vi "CardStatusInitial.vi"(7 "Action":enum16{"Initial", "Write", "Read", "Release"}(ring)=enum."Release", 9 "DataIn":T2, 10 "CardNumber":i32, 11 "IOCard":refnum<vi>) -> (2 "CardStatus":T1(array[cluster]))   [LabVIEW 2019, in "IOCard.lvclass"]
uses:
  IOCard.lvclass
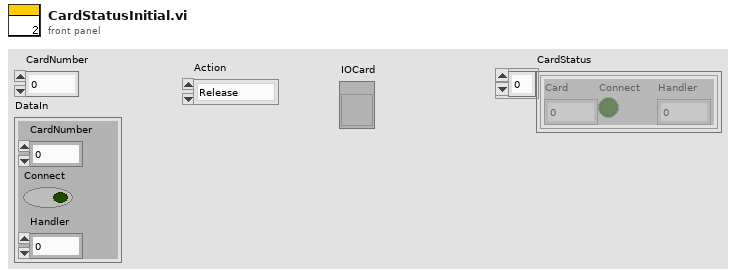
[diagram p1: front panel]
types:
  T1 = cluster{"Card":i32, "Connect":bool, "Handler":i32}[]
  T2 = cluster{"CardNumber":i32, "Connect":bool, "Handler":i32}
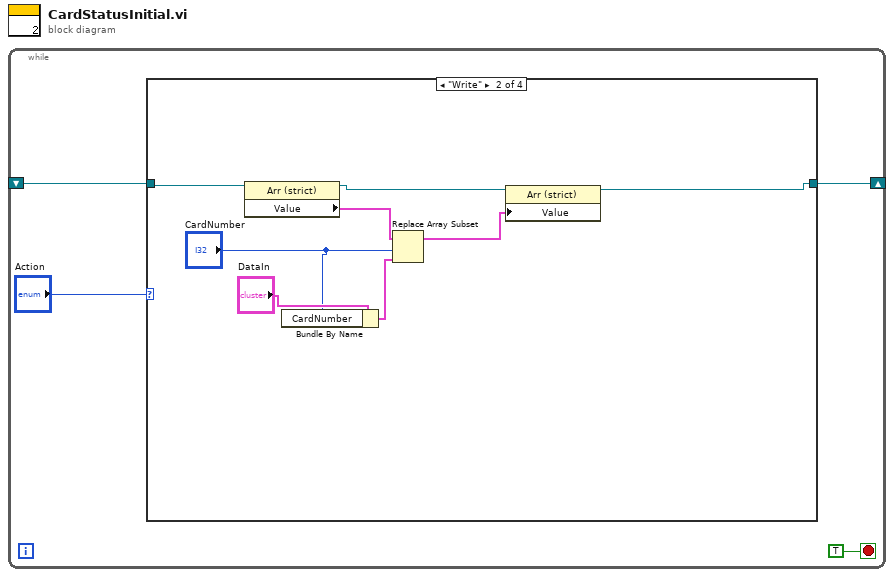
[diagram p0: block diagram]
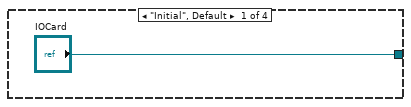
[diagram p2: hidden frame]
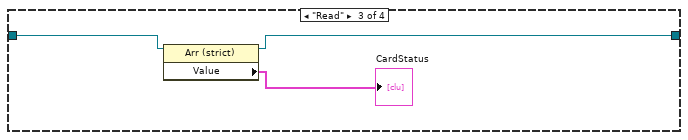
[diagram p3: hidden frame]
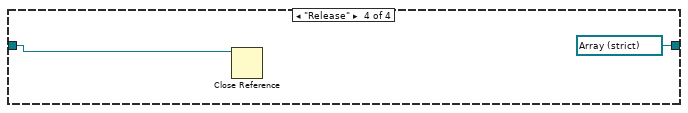
[diagram p4: hidden frame]
diagram:
  n1 = while {
    shift-right: [w4] -> _
    shift-left: _ -> [w3]
    stop <- TRUE stop-if-true
    n2 = case shown="\"Write\"" "Action" {
      tunnel: ["IOCard" w9 w15 refnum<vi> refnum ("IOCard")] -> w4
      tunnel: w3 -> [_ w13 w16 w18]
      frame "Initial", Default {
      }
      frame "Write" {
        n3 = property class="Arr (strict)"(reference=w13) -> (reference out=w11:refnum<vi>, "Value"=w12:T1)  [unwired: 1 in, 1 out]
        n4 = Bundle By Name(cluster="DataIn", "CardNumber"="CardNumber") -> (w6:T2)
        n5 = Replace Array Subset(array=w12, new element=w6, index="CardNumber") -> (w10:T1)
        n6 = property class="Arr (strict)"(reference=w11, "Value"=w10) -> (reference out=w9:refnum<vi>)  [unwired: 1 in, 1 out]
      }
      frame "Read" {
        n7 = property class="Arr (strict)"(reference=w16) -> (reference out=w15:refnum<vi>, "Value"=→"CardStatus":T1)  [unwired: 1 in, 1 out]
      }
      frame "Release" {
        n8 = Close Reference(reference=w18) -> ()  [unwired: 1 in, 1 out]
      }
    }
  }
